vi "get_immersion.vi"(8 "error in (no error)":errorcluster, 11 "GenericObjective in":refnum<class "GenericObjective.lvclass">) -> (0 "error out":errorcluster, 2 "Immersion":T1, 3 "GenericObjective out":refnum<class "GenericObjective.lvclass">)   [LabVIEW 2010, in "GenericObjective.lvclass"]
uses:
  GenericObjective.lvclass
  immersion_enum.ctl
  GenericObjective.lvclass/GenericObjective.ctl
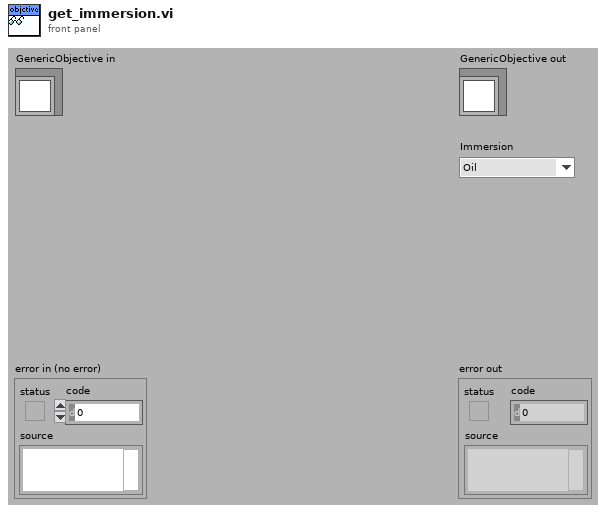
[diagram p1: front panel]
types:
  T1 = typedef "GenericObjective.lvclass/immersion_enum.ctl" = enum16{"Oil", "Water", "WaterDipping", "Air", "Multi", "Glycerol", "Other", "Unknown"}
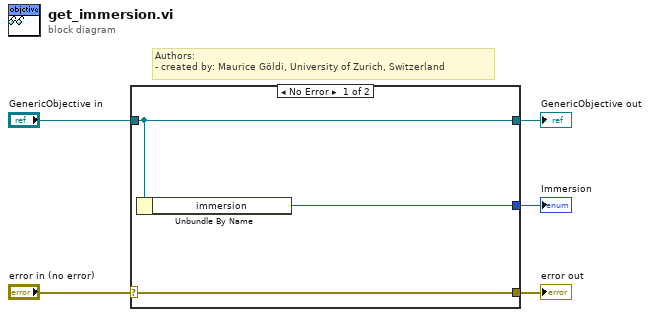
[diagram p0: block diagram]
diagram:
  # "Authors: \n- created by: Maurice Göldi, University of Zurich, Switzerland"
  n1 = case shown="No Error" "error in (no error)" {
    selector: "error in (no error)" -> [w8 w9]
    tunnel: [w8 w9] -> w4
    tunnel: [w7 w10] -> w2
    tunnel: "GenericObjective in" -> [w7 w10]
    tunnel: [w6 _] -> w1
    frame No Error {
      n2 = Unbundle By Name(w7) -> ("immersion"=w6:T1)
    }
    frame Error {
    }
  }
  "error out" <- w4
  "GenericObjective out" <- w2
  "Immersion" <- w1
